vi "ChangeFileName.vi"(2 "input par":T1={"Folder"=path "", "Name"="trace", "Ext"="ccd"}) -> (0 "output par":T1={"Folder"=path "", "Name"="trace", "Ext"="ccd"}, 1 "OK ?":bool)   [LabVIEW 2011]
doc: "Prompt User to enter new file name while using the initial values for both the path and the name as starting points."
panel:
  in  "Cancel Button":bool
  in  "OK Button":bool
  in  "Ext":string="ccd"
  in  "Name":string="trace"
  in  "Folder":path
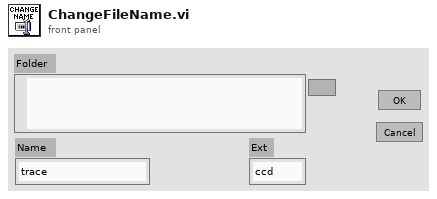
[diagram p1: front panel]
types:
  T1 = cluster{"Folder":path, "Name":string, "Ext":string}
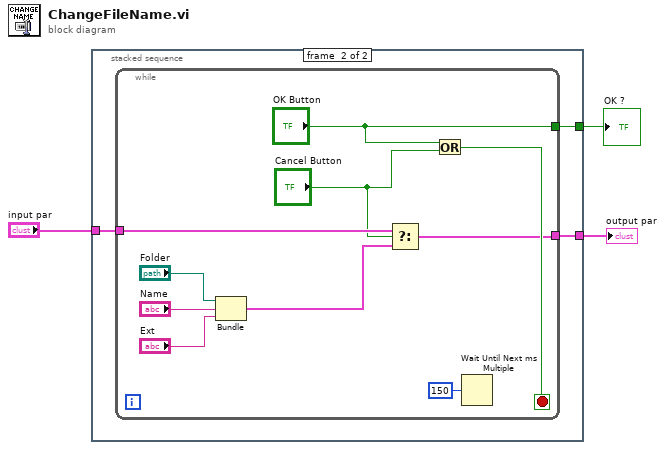
[diagram p0: block diagram]
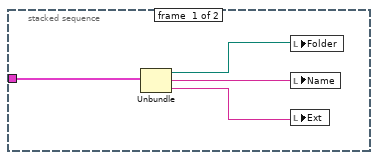
[diagram p2: hidden frame]
diagram:
  n1 = stacked-sequence {
    tunnel: "input par" -> [w7 w10]
    tunnel: [_ w9] -> w2
    tunnel: [_ w8] -> w1
    frame #0 {
      n2 = Unbundle(w7) -> ("Folder"=w6:path, "Name"=w5:string, "Ext"=w4:string)
      n3 = local write "Folder"(w6) -> ()
      n4 = local write "Name"(w5) -> ()
      n5 = local write "Ext"(w4) -> ()
    }
    frame #1 {
      n6 = while {
        tunnel: w10 -> [w15]
        tunnel: [w12] -> w9
        tunnel: ["OK Button"] -> w8
        stop <- w16 stop-if-true
        n7 = Bundle("Folder"="Folder", "Name"="Name", "Ext"="Ext") -> (w13:T1)  [unwired: 1 in]
        n8 = Select(t=w15, s="Cancel Button", f=w13) -> (s? t:f=w12:T1)
        n9 = Or(x="OK Button", y="Cancel Button") -> (x .or. y?=w16:bool)
        n10 = Wait Until Next ms Multiple(millisecond multiple=u32 150) -> ()  [unwired: 1 out]
      }
    }
  }
  "output par" <- w2
  "OK ?" <- w1
